vi "Pause.vi"(8 "error in (no error)":errorcluster, 11 "Channel in":refnum<data-value>) -> (0 "error out":errorcluster, 3 "Channel out":refnum<data-value>)   [LabVIEW 2020, in "G-Audio.lvlib" / "Channel.lvclass"]
uses:
  Channel.lvclass
  Channel.lvclass/Channel.ctl
  Channel State.ctl
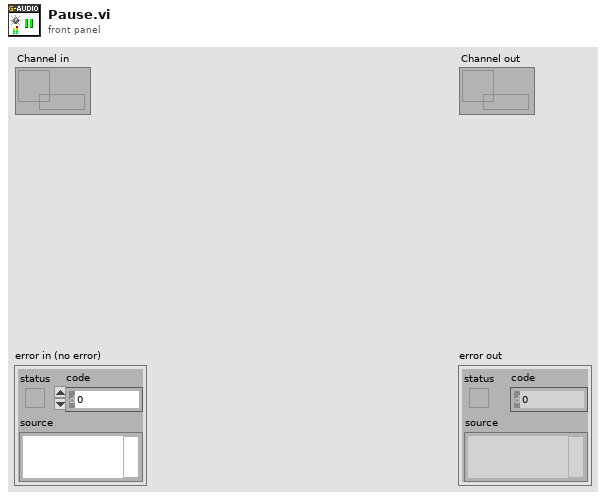
[diagram p1: front panel]
types:
  T1 = typedef "G-Audio.lvlib/Channel.lvclass/Channel State.ctl" = enum16{"Empty", "Loading", "Stopped", "Paused", "Playing", "Retrigger"}
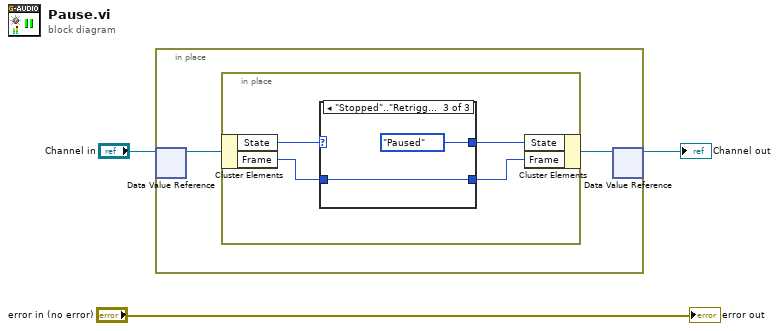
[diagram p0: block diagram]
diagram:
  n1 = in-place {
    n2 = in-place-dvr #1("Channel in") -> (w5:refnum<class "Channel.lvclass">)  [unwired: 1 out]
    n3 = in-place {
      n4 = in-place-cluster #2(w5) -> ("State"=w9:T1, "Frame"=w8:u64)
      n5 = case shown="\"Stopped\"..\"Retrigger\"" w9 {
        selector: w9 -> [w11 w13 _]
        tunnel: [w11 w13 Channel_State."Paused" ("data value")] -> w7
        tunnel: [w10 w12 w14] -> w6
        tunnel: w8 -> [w10 w12 w14]
        frame "Empty", Default {
        }
        frame "Loading" {
        }
        frame "Stopped".."Retrigger" {
        }
      }
      n6 = in-place-cluster #2("State"=w7, "Frame"=w6) -> (w4:refnum<class "Channel.lvclass">)
    }
    n7 = in-place-dvr #1(w4) -> (→"Channel out":refnum<data-value>)  [unwired: 1 out]
  }
  "error out" <- "error in (no error)"
